vi "Cycle_Diag_Table_Read_FL24_Dryer.vi"(7 "ERD Data In":T3[](array[typedef]) {"ERD Number" format="%.0x"}, 11 "error in (no error)":errorcluster) -> (2 "Cycle Buffer Status":T2, 3 "Diag Cycle String Out":string[][](array[string]), 15 "error out":errorcluster)   [LabVIEW 2016]
uses:
  Common/LabVIEW GEA2 Toolkit/LabVIEW_GEA2_Toolkit.lvlibp/type defs/ERD Read Data Out.ctl
  type defs/Cycle_Diag_Buffer_Status.ctl
  type defs/Cycle_Diag.ctl
  Common/LabVIEW GEA2 Toolkit/LabVIEW_GEA2_Toolkit.lvlibp
panel:
  out "Cycle Diag Array Out":T1[](array[typedef])
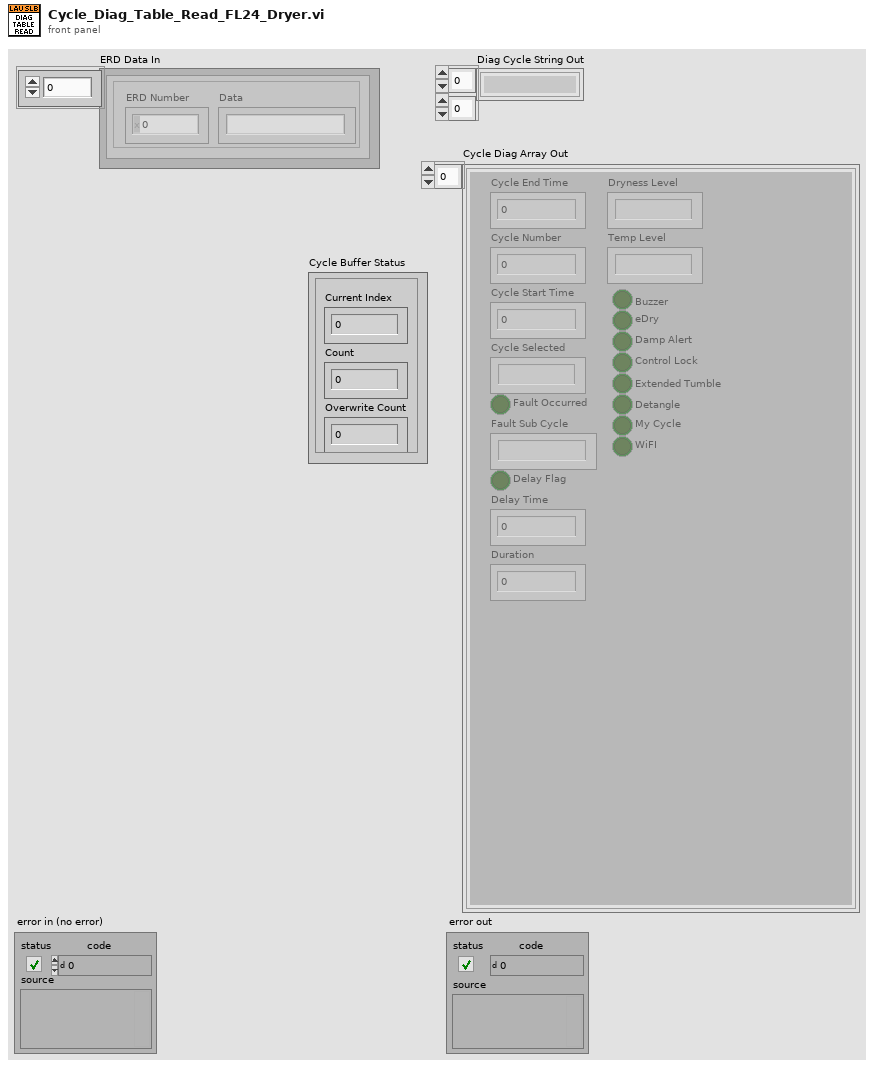
[diagram p1: front panel]
types:
  T1 = typedef "Cycle_Diag.ctl" = cluster{"Cycle End Time":u32, "Cycle Number":u32, "Cycle Start Time":u32, "Fault Sub Cycle":string, "Dryness Level":string, "Temp Level":string, "Fault Occurred":bool, "Delay Flag":bool, "Cycle Selected":string, "Buzzer":bool, "eDry":bool, "Damp Alert":bool, "Control Lock":bool, "Extended Tumble":bool, "Detangle":bool, "My Cycle":bool, "WiFI":bool, "Delay Time":u8, "Duration":u8}
  T2 = typedef "Cycle_Diag_Buffer_Status.ctl" = cluster{"Current Index":u16, "Count":u16, "Overwrite Count":u16}
  T3 = typedef "LabVIEW_GEA2_Toolkit.lvlibp/ERD Read Data Out.ctl" = cluster{"ERD Number":u16, "Data":string}
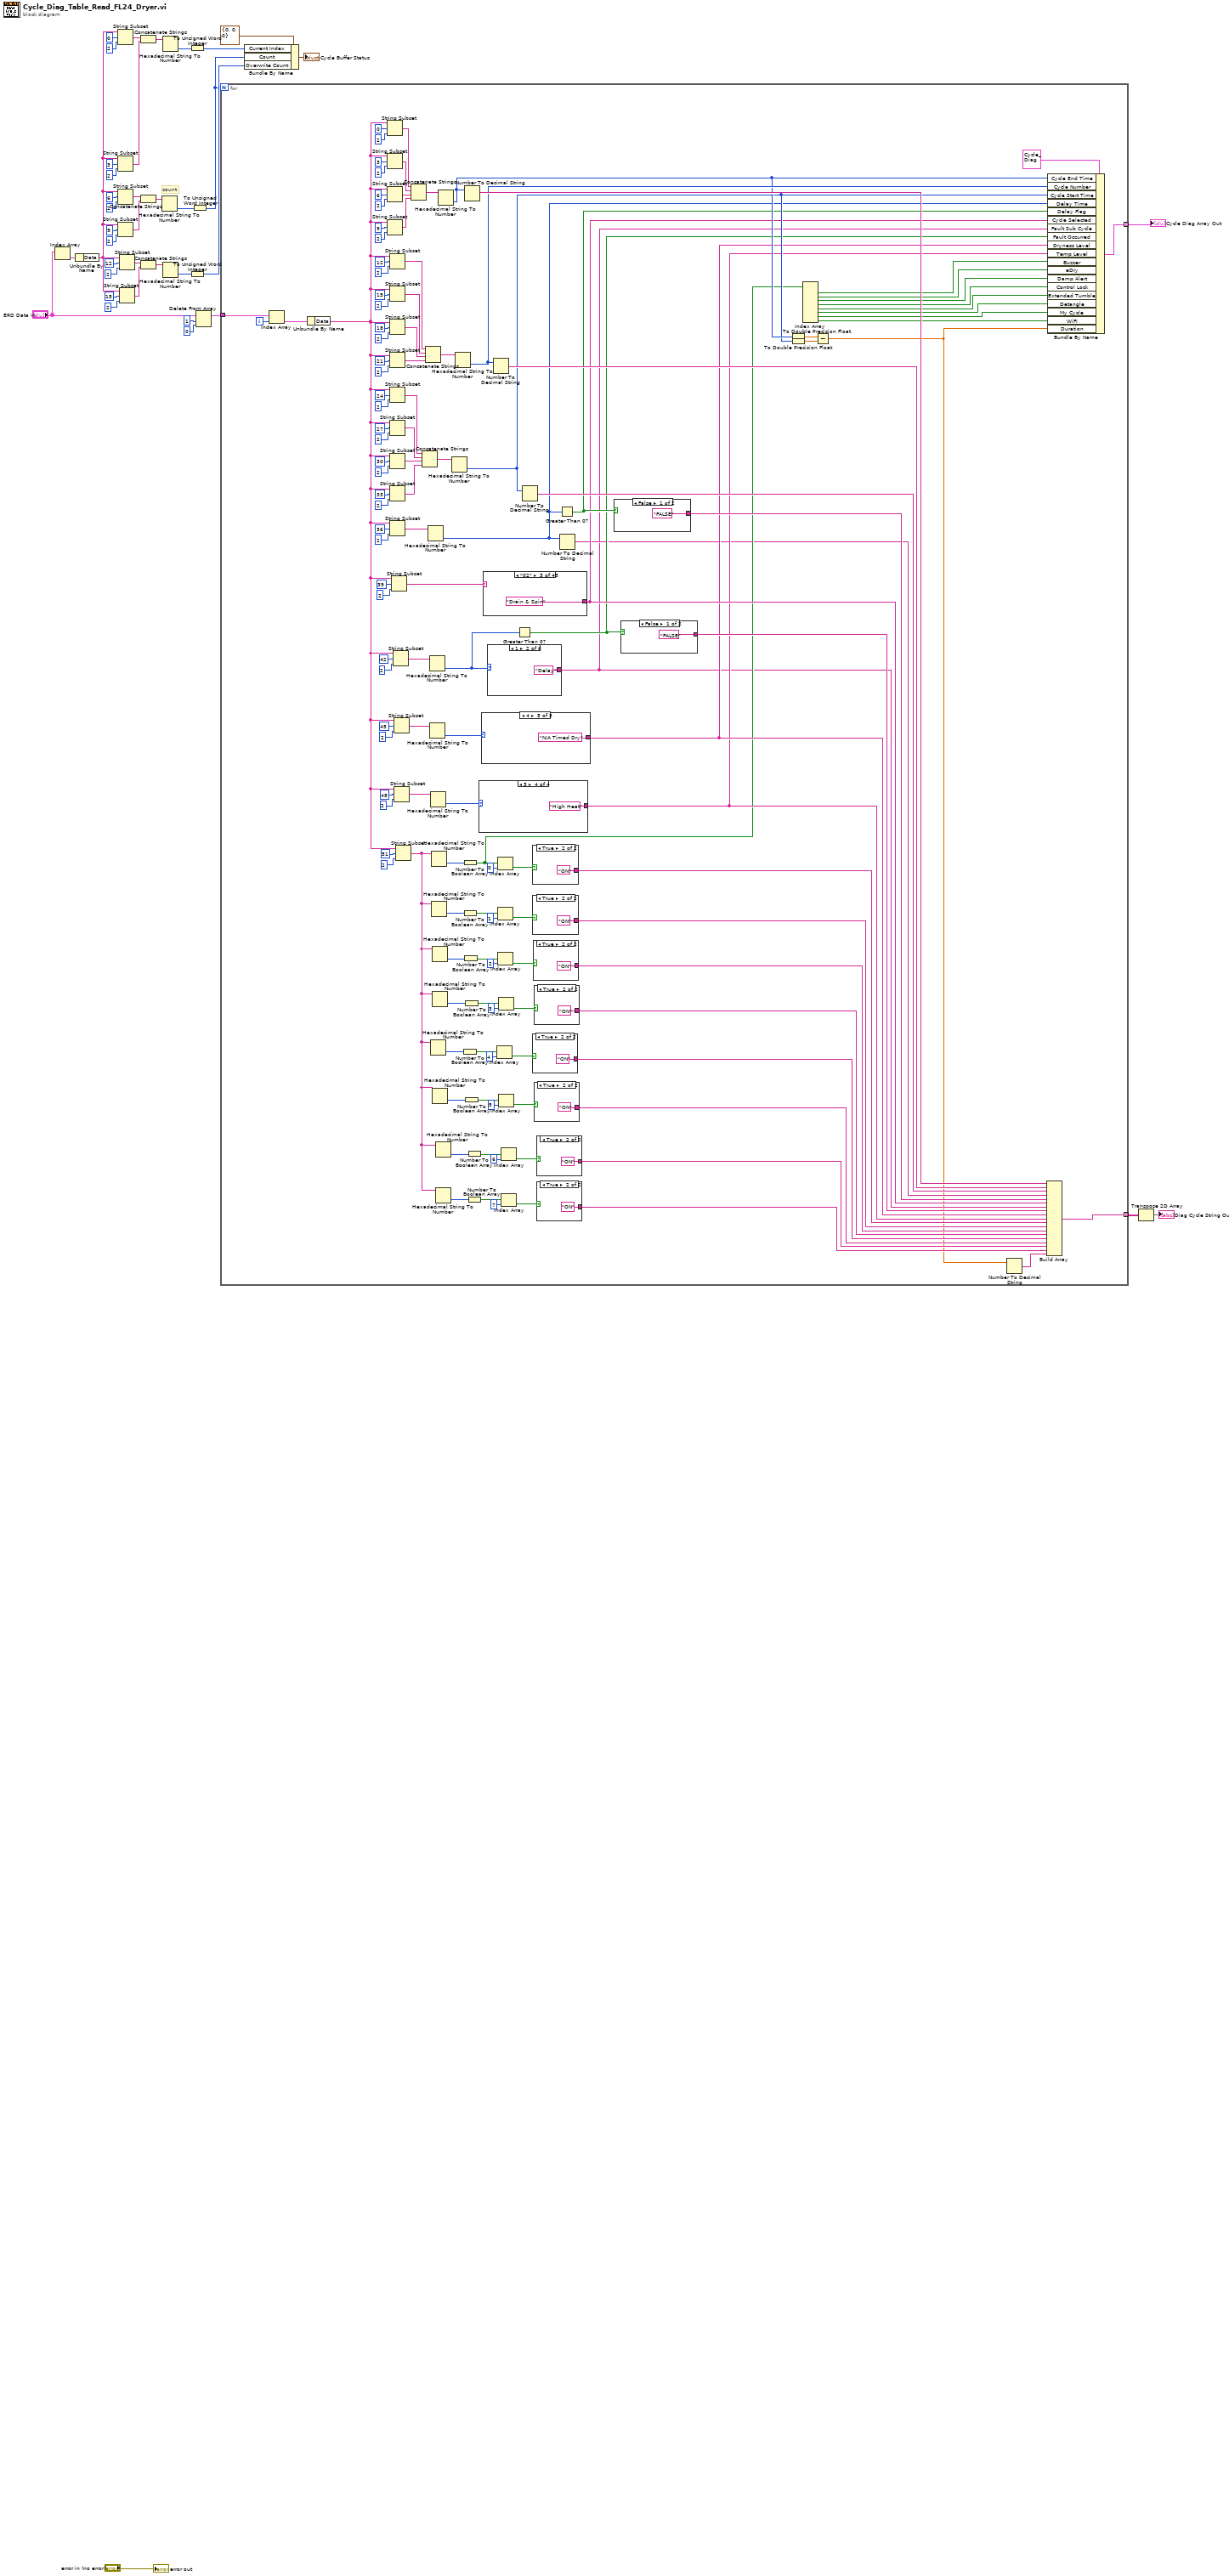
[diagram p0: block diagram]
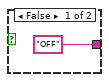
[diagram p2: hidden frame]
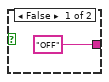
[diagram p3: hidden frame]
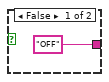
[diagram p4: hidden frame]
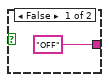
[diagram p5: hidden frame]
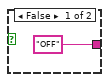
[diagram p6: hidden frame]
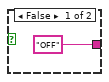
[diagram p7: hidden frame]
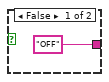
[diagram p8: hidden frame]
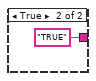
[diagram p9: hidden frame]
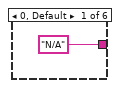
[diagram p10: hidden frame]
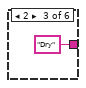
[diagram p11: hidden frame]
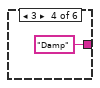
[diagram p12: hidden frame]
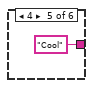
[diagram p13: hidden frame]
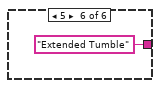
[diagram p14: hidden frame]
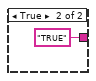
[diagram p15: hidden frame]
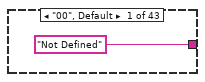
[diagram p16: hidden frame]
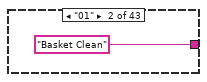
[diagram p17: hidden frame]
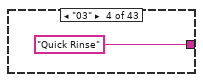
[diagram p18: hidden frame]
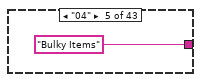
[diagram p19: hidden frame]
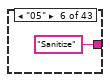
[diagram p20: hidden frame]
diagram:
  # "count"
  n1 = Index Array(array="ERD Data In") -> (element=w32:T3)  [unwired: 1 in]
  n2 = Unbundle By Name(w32) -> ("Data"=w12:string)
  n3 = String Subset(string=w12, offset (0)=0, length (rest)=2 ("length (rest)")) -> (substring=w21:string)
  n4 = String Subset(string=w12, offset (0)=3, length (rest)=2 ("length (rest)")) -> (substring=w22:string)
  n5 = String Subset(string=w12, offset (0)=6, length (rest)=2 ("length (rest)")) -> (substring=w36:string)
  n6 = String Subset(string=w12, offset (0)=9, length (rest)=2 ("length (rest)")) -> (substring=w35:string)
  n7 = String Subset(string=w12, offset (0)=12, length (rest)=2 ("length (rest)")) -> (substring=w23:string)
  n8 = String Subset(string=w12, offset (0)=15, length (rest)=2 ("length (rest)")) -> (substring=w24:string)
  n9 = Concatenate Strings(w21, w22) -> (w25:string)
  n10 = Concatenate Strings(w36, w35) -> (w34:string)
  n11 = Concatenate Strings(w23, w24) -> (w26:string)
  n12 = Hexadecimal String To Number(string=w34) -> (number=w33:u32)  [unwired: 2 in, 1 out]
  n13 = Hexadecimal String To Number(string=w25) -> (number=w27:u32)  [unwired: 2 in, 1 out]
  n14 = Hexadecimal String To Number(string=w26) -> (number=w28:u32)  [unwired: 2 in, 1 out]
  n15 = To Unsigned Word Integer(number=w27) -> (unsigned 16bit integer=w29:u16)
  n16 = To Unsigned Word Integer(number=w28) -> (unsigned 16bit integer=w30:u16)
  n17 = To Unsigned Word Integer(number=w33) -> (unsigned 16bit integer=w11:u16)
  n18 = Delete From Array(array="ERD Data In", length=1, index=0) -> (array with subset deleted=w8:T3[])  [unwired: 1 out]
  n19 = for {
    N: w11 -> [_]
    tunnel: w8 -> [w133]
    tunnel: [w130] -> w1 mode=indexing
    tunnel: [w129] -> w4 mode=indexing
    i -> [w132]
    n20 = Index Array(array=w133, index=w132) -> (element=w131:T3)
    n21 = Unbundle By Name(w131) -> ("Data"=w106:string)
    n22 = String Subset(string=w106, offset (0)=0, length (rest)=2 ("length (rest)")) -> (substring=w148:string)
    n23 = String Subset(string=w106, offset (0)=3, length (rest)=2 ("length (rest)")) -> (substring=w147:string)
    n24 = String Subset(string=w106, offset (0)=6, length (rest)=2 ("length (rest)")) -> (substring=w146:string)
    n25 = String Subset(string=w106, offset (0)=9, length (rest)=2 ("length (rest)")) -> (substring=w145:string)
    n26 = String Subset(string=w106, offset (0)=12, length (rest)=2 ("length (rest)")) -> (substring=w143:string)
    n27 = String Subset(string=w106, offset (0)=15, length (rest)=2 ("length (rest)")) -> (substring=w142:string)
    n28 = String Subset(string=w106, offset (0)=18, length (rest)=2 ("length (rest)")) -> (substring=w141:string)
    n29 = String Subset(string=w106, offset (0)=21, length (rest)=2 ("length (rest)")) -> (substring=w140:string)
    n30 = String Subset(string=w106, offset (0)=24, length (rest)=2 ("length (rest)")) -> (substring=w138:string)
    n31 = String Subset(string=w106, offset (0)=27, length (rest)=2 ("length (rest)")) -> (substring=w137:string)
    n32 = String Subset(string=w106, offset (0)=30, length (rest)=2 ("length (rest)")) -> (substring=w136:string)
    n33 = String Subset(string=w106, offset (0)=33, length (rest)=2 ("length (rest)")) -> (substring=w135:string)
    n34 = String Subset(string=w106, offset (0)=36, length (rest)=2 ("length (rest)")) -> (substring=w101:string)
    n35 = String Subset(string=w106, offset (0)=39, length (rest)=2 ("length (rest)")) -> (substring=w97:string)
    n36 = String Subset(string=w106, offset (0)=42, length (rest)=2 ("length (rest)")) -> (substring=w121:string)
    n37 = String Subset(string=w106, offset (0)=45, length (rest)=2 ("length (rest)")) -> (substring=w116:string)
    n38 = String Subset(string=w106, offset (0)=48, length (rest)=2 ("length (rest)")) -> (substring=w114:string)
    n39 = String Subset(string=w106, offset (0)=51, length (rest)=2 ("length (rest)")) -> (substring=w58:string)
    n40 = Concatenate Strings(w148, w147, w146, w145) -> (w144:string)
    n41 = Concatenate Strings(w138, w137, w136, w135) -> (w134:string)
    n42 = Concatenate Strings(w143, w142, w141, w140) -> (w139:string)
    n43 = Hexadecimal String To Number(string=w101) -> (number=w100:u32)  [unwired: 2 in, 1 out]
    n44 = Hexadecimal String To Number(string=w121) -> (number=w95:u32)  [unwired: 2 in, 1 out]
    n45 = Hexadecimal String To Number(string=w116) -> (number=w115:u32)  [unwired: 2 in, 1 out]
    n46 = Hexadecimal String To Number(string=w114) -> (number=w91:u32)  [unwired: 2 in, 1 out]
    n47 = Hexadecimal String To Number(string=w58) -> (number=w74:u32)  [unwired: 2 in, 1 out]
    n48 = Hexadecimal String To Number(string=w58) -> (number=w109:u32)  [unwired: 2 in, 1 out]
    n49 = Hexadecimal String To Number(string=w58) -> (number=w86:u32)  [unwired: 2 in, 1 out]
    n50 = Hexadecimal String To Number(string=w58) -> (number=w85:u32)  [unwired: 2 in, 1 out]
    n51 = Hexadecimal String To Number(string=w58) -> (number=w75:u32)  [unwired: 2 in, 1 out]
    n52 = Hexadecimal String To Number(string=w58) -> (number=w67:u32)  [unwired: 2 in, 1 out]
    n53 = Hexadecimal String To Number(string=w58) -> (number=w66:u32)  [unwired: 2 in, 1 out]
    n54 = Hexadecimal String To Number(string=w58) -> (number=w59:u32)  [unwired: 2 in, 1 out]
    n55 = Hexadecimal String To Number(string=w144) -> (number=w105:u32)  [unwired: 2 in, 1 out]
    n56 = Hexadecimal String To Number(string=w134) -> (number=w104:u32)  [unwired: 2 in, 1 out]
    n57 = Hexadecimal String To Number(string=w139) -> (number=w125:u32)  [unwired: 2 in, 1 out]
    n58 = Number To Boolean Array(number=w74) -> (Boolean array=w73:bool[])
    n59 = Number To Boolean Array(number=w109) -> (Boolean array=w52:bool[])
    n60 = Number To Boolean Array(number=w86) -> (Boolean array=w87:bool[])
    n61 = Number To Boolean Array(number=w85) -> (Boolean array=w84:bool[])
    n62 = Number To Boolean Array(number=w75) -> (Boolean array=w76:bool[])
    n63 = Number To Boolean Array(number=w67) -> (Boolean array=w68:bool[])
    n64 = Number To Decimal String(number=w105) -> (decimal integer string=w127:string)  [unwired: 1 in]
    n65 = Number To Boolean Array(number=w66) -> (Boolean array=w65:bool[])
    n66 = Number To Boolean Array(number=w59) -> (Boolean array=w60:bool[])
    n67 = case shown="3" w91 {
      tunnel: ["No Heat" "Low Heat" "Medium Heat" "High Heat"] -> w90
      frame 0, Default {
      }
      frame 1 {
      }
      frame 2 {
      }
      frame 3 {
      }
    }
    n68 = case shown="4" w115 {
      tunnel: ["Damp" "Less Dry" "Dry" "Extra Dry" "N/A Timed Dry"] -> w92
      frame 0, Default {
      }
      frame 1 {
      }
      frame 2 {
      }
      frame 3 {
      }
      frame 4 {
      }
    }
    n69 = case shown="\"02\"" w97 {
      tunnel: ["Not Defined" "Basket Clean" "Drain & Spin" "Quick Rinse" "Bulky Items" "Sanitize" "Towels & Sheets" "Steam Refresh" "Normal/Mixed" "Whites" "Dark Colors" "Jeans" "Hand Wash" "Delicates" "Speed Wash" "Heavy Duty" "Allergen" "Power Clean" "Rinse & Spin" "Single Item" "Colors" "Cold Wash" "Water on Demand" "Tub Clean" "Casuals w/ Steam" "Stain Wash w/ Steam" "Cottons" "Easy Care" "Active Wear" "Timed Dry" "Dewrinkle" "Air Fluff" "Steam Refresh" "Steam Dewrinkle" "Speed Dry" "Mixed" "Quick Dry" "Casuals" "Warm Up" "Energy Saver" "Antibacterial" "Rack Dry" "Baby Care"] -> w96
      frame "00", Default {
      }
      frame "01" {
      }
      frame "02" {
      }
      frame "03" {
      }
      frame "04" {
      }
      frame "05" {
      }
      frame "06" {
      }
      frame "07" {
      }
      frame "08" {
      }
      frame "09" {
      }
      frame "0A" {
      }
      frame "0B" {
      }
      frame "0C" {
      }
      frame "0D" {
      }
      frame "0E" {
      }
      frame "0F" {
      }
      frame "10" {
      }
      frame "11" {
      }
      frame "12" {
      }
      frame "13" {
      }
      frame "14" {
      }
      frame "15" {
      }
      frame "16" {
      }
      frame "17" {
      }
      frame "18" {
      }
      frame "19" {
      }
      frame "80" {
      }
      frame "81" {
      }
      frame "82" {
      }
      frame "83" {
      }
      frame "84" {
      }
      frame "85" {
      }
      frame "86" {
      }
      frame "87" {
      }
      frame "88" {
      }
      frame "89" {
      }
      frame "8A" {
      }
      frame "8B" {
      }
      frame "8C" {
      }
      frame "8D" {
      }
      frame "8E" {
      }
      frame "8F" {
      }
      frame "90" {
      }
    }
    n70 = case shown="1" w95 {
      tunnel: ["N/A" "Delay" "Dry" "Damp" "Cool" "Extended Tumble"] -> w42
      frame 0, Default {
      }
      frame 1 {
      }
      frame 2 {
      }
      frame 3 {
      }
      frame 4 {
      }
      frame 5 {
      }
    }
    n71 = Number To Decimal String(number=w125) -> (decimal integer string=w126:string)  [unwired: 1 in]
    n72 = Index Array(array=w73, index=4) -> (element=w71:bool)
    n73 = Index Array(array=w52, index=0) -> (element=w107:bool)
    n74 = Index Array(array=w87, index=1) -> (element=w89:bool)
    n75 = Index Array(array=w84, index=2) -> (element=w82:bool)
    n76 = Index Array(array=w76, index=3) -> (element=w78:bool)
    n77 = Index Array(array=w68, index=5) -> (element=w70:bool)
    n78 = Index Array(array=w65, index=6) -> (element=w63:bool)
    n79 = Index Array(array=w60, index=7) -> (element=w62:bool)
    n80 = Greater Than 0?(x=w95) -> (x > 0?=w94:bool)
    n81 = Number To Decimal String(number=w104) -> (decimal integer string=w124:string)  [unwired: 1 in]
    n82 = case shown="True" w71 {
      tunnel: ["OFF" "ON"] -> w56
      frame False {
      }
      frame True {
      }
    }
    n83 = case shown="True" w107 {
      tunnel: ["OFF" "ON"] -> w81
      frame False {
      }
      frame True {
      }
    }
    n84 = case shown="True" w89 {
      tunnel: ["OFF" "ON"] -> w80
      frame False {
      }
      frame True {
      }
    }
    n85 = case shown="True" w82 {
      tunnel: ["OFF" "ON"] -> w79
      frame False {
      }
      frame True {
      }
    }
    n86 = case shown="True" w78 {
      tunnel: ["OFF" "ON"] -> w57
      frame False {
      }
      frame True {
      }
    }
    n87 = case shown="True" w70 {
      tunnel: ["OFF" "ON"] -> w55
      frame False {
      }
      frame True {
      }
    }
    n88 = case shown="True" w63 {
      tunnel: ["OFF" "ON"] -> w54
      frame False {
      }
      frame True {
      }
    }
    n89 = case shown="True" w62 {
      tunnel: ["OFF" "ON"] -> w53
      frame False {
      }
      frame True {
      }
    }
    n90 = Greater Than 0?(x=w100) -> (x > 0?=w99:bool)
    n91 = Number To Decimal String(number=w100) -> (decimal integer string=w43:string)  [unwired: 1 in]
    n92 = case shown="False" w99 {
      tunnel: ["FALSE" "TRUE"] -> w98
      frame False {
      }
      frame True {
      }
    }
    n93 = case shown="False" w94 {
      tunnel: ["FALSE" "TRUE"] -> w93
      frame False {
      }
      frame True {
      }
    }
    n94 = To Double Precision Float(number=w105) -> (double precision float=w103:dbl)
    n95 = To Double Precision Float(number=w104) -> (double precision float=w102:dbl)
    n96 = Index Array(array=w52) -> (element #1=w51:bool, element #2=w50:bool, element #3=w49:bool, element #4=w48:bool, element #5=w47:bool, element #6=w46:bool, element #7=w45:bool, element #8=w44:bool)  [unwired: 8 in]
    n97 = Subtract(x=w103, y=w102) -> (x-y=w41:dbl)
    n98 = Number To Decimal String(number=w41) -> (decimal integer string=w40:string)  [unwired: 1 in]
    n99 = Build Array(w127, w126, w124, w43, w98, w96, w42, w93, w92, w90, w81, w80, w79, w57, w56, w55, w54, w53, w40) -> (w129:string[])
    n100 = Bundle By Name(cluster=T1 {"Cycle End Time"=0, "Cycle Number"=0, "Cycle Start Time"=0, "Fault Sub Cycle"="", "Dryness Level"="", "Temp Level"="", "Fault Occurred"=FALSE, "Delay Flag"=FALSE, "Cycle Selected"="", "Buzzer"=FALSE, "eDry"=FALSE, "Damp Alert"=FALSE, "Control Lock"=FALSE, "Extended Tumble"=FALSE, "Detangle"=FALSE, "My Cycle"=FALSE, "WiFI"=FALSE, "Delay Time"=0, "Duration"=0} ("Cycle History Diagnostics"), "Cycle End Time"=w105, "Cycle Number"=w125, "Cycle Start Time"=w104, "Delay Time"=w100, "Delay Flag"=w99, "Cycle Selected"=w96, "Fault Sub Cycle"=w42, "Fault Occurred"=w94, "Dryness Level"=w92, "Temp Level"=w90, "Buzzer"=w51, "eDry"=w50, "Damp Alert"=w49, "Control Lock"=w48, "Extended Tumble"=w47, "Detangle"=w46, "My Cycle"=w45, "WiFI"=w44, "Duration"=w41) -> (w130:T1)
  }
  "Cycle Diag Array Out" <- w1
  n101 = Bundle By Name(cluster=T2 {"Current Index"=0, "Count"=0, "Overwrite Count"=0} ("Cycle Buffer Status"), "Current Index"=w29, "Count"=w11, "Overwrite Count"=w30) -> (→"Cycle Buffer Status":T2)
  n102 = Transpose 2D Array(2D array=w4) -> (transposed array=→"Diag Cycle String Out":string[][])
  "error out" <- "error in (no error)"
